vi "Self Actor Decorator.vi"(10 "Self Actor":refnum<class "LVCAM.lvclass">, 11 "Write Actor in":refnum<class "Self Actor Decorator.lvclass">) -> (3 "Write Actor out":refnum<class "Self Actor Decorator.lvclass">)   [LabVIEW 2021, in "LVCAM.lvlib" / "Self Actor Decorator.lvclass"]
uses:
  Self Actor Decorator.lvclass
  LVCAM/LVCAM.lvclass
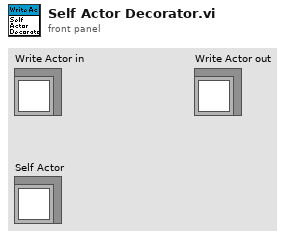
[diagram p1: front panel]
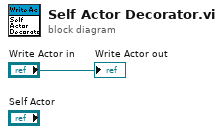
[diagram p0: block diagram]
diagram:
  "Write Actor out" <- "Write Actor in"
